vi "convert lat and long.vi"(2 "GPS Data":T1) -> (5 "Latitude":dbl, 6 "Longtitude":dbl)   [LabVIEW 2012]
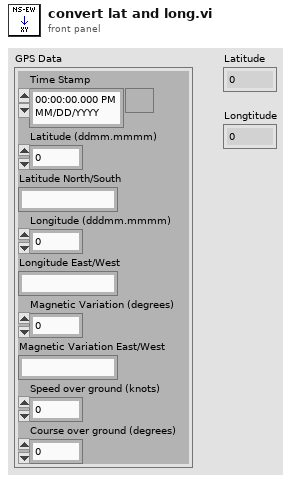
[diagram p1: front panel]
types:
  T1 = cluster{"Time Stamp":timestamp, "Latitude (ddmm.mmmm)":dbl, "Latitude North/South":string, "Longitude (dddmm.mmmm)":dbl, "Longitude East/West":string, "Magnetic Variation (degrees)":dbl, "Magnetic Variation East/West":string, "Speed over ground (knots)":dbl, "Course over ground (degrees)":dbl}
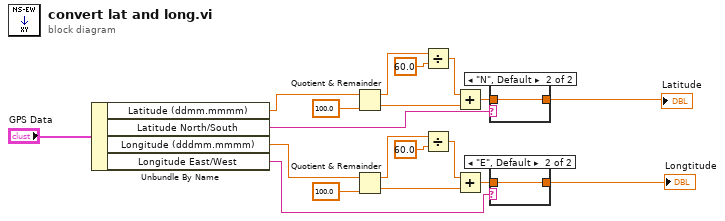
[diagram p0: block diagram]
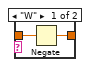
[diagram p2: hidden frame]
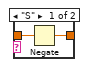
[diagram p3: hidden frame]
diagram:
  n1 = Unbundle By Name("GPS Data") -> ("Latitude (ddmm.mmmm)"=w13:dbl, "Latitude North/South"=w14:string, "Longitude (dddmm.mmmm)"=w15:dbl, "Longitude East/West"=w16:string)
  n2 = Quotient & Remainder(x=w13, y=100.0) -> (x-y*floor(x/y)=w2:dbl, floor(x/y)=w4:dbl)
  n3 = Quotient & Remainder(x=w15, y=100.0) -> (x-y*floor(x/y)=w11:dbl, floor(x/y)=w9:dbl)
  n4 = Divide(x=w2, y=60.0) -> (x/y=w5:dbl)
  n5 = Divide(x=w11, y=60.0) -> (x/y=w8:dbl)
  n6 = Add(x=w5, y=w4) -> (x+y=w6:dbl)
  n7 = Add(x=w8, y=w9) -> (x+y=w7:dbl)
  n8 = case shown="\"N\", Default" w14 {
    tunnel: w6 -> [w21 w22]
    tunnel: [w20 w22] -> w17
    frame "S" {
      n9 = Negate(x=w21) -> (-x=w20:dbl)
    }
    frame "N", Default {
    }
  }
  "Latitude" <- w17
  n10 = case shown="\"E\", Default" w16 {
    tunnel: w7 -> [w24 w25]
    tunnel: [w23 w25] -> w18
    frame "W" {
      n11 = Negate(x=w24) -> (-x=w23:dbl)
    }
    frame "E", Default {
    }
  }
  "Longtitude" <- w18
